vi "Lookup Target ID.vi"(8 "error in (no error)":errorcluster, 10 "Target Name":string, 11 "VolatusAPI in":refnum<class "VolatusAPI.lvclass">) -> (0 "error out":errorcluster, 2 "Target ID":u32, 3 "VolatusAPI out":refnum<class "VolatusAPI.lvclass">)   [LabVIEW 2020, in "Volatus.lvlib" / "VolatusAPI.lvclass"]
uses:
  VolatusAPI.lvclass
  VolatusAPI.lvclass/VolatusAPI.ctl
  VolatusConfig/Node/Node.lvclass
  VolatusConfig/Cluster/Cluster.lvclass
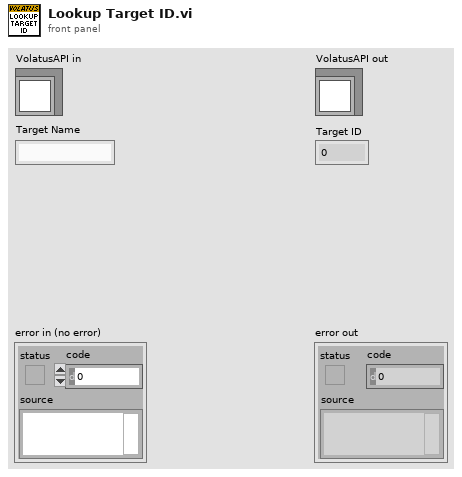
[diagram p1: front panel]
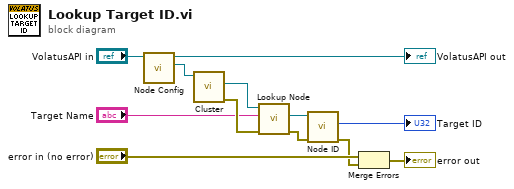
[diagram p0: block diagram]
diagram:
  n1 = call "Node Config.vi"("VolatusAPI in"="VolatusAPI in") -> ("Node Config"=w8:refnum<class "Node.lvclass">, "VolatusAPI out"=→"VolatusAPI out":refnum<class "VolatusAPI.lvclass">)  [unwired: 9 in]
  n2 = call "Cluster.vi"("Node in"=w8) -> ("error out"=w12:errorcluster, "Cluster"=w7:refnum<class "Cluster.lvclass">)  [unwired: 8 in, 1 out]
  n3 = call "Lookup Node.vi"("error in (no error)"=w12, "Node Name"="Target Name", "Cluster in"=w7) -> ("error out"=w4:errorcluster, "Node"=w5:refnum<class "Node.lvclass">)  [unwired: 6 in, 1 out]
  n4 = call "Node ID.vi"("error in (no error)"=w4, "Node in"=w5) -> ("error out"=w1:errorcluster, "Node ID"=→"Target ID":u32)  [unwired: 7 in, 1 out]
  n5 = Merge Errors("error in (no error)", w1) -> (→"error out":errorcluster)
